vi "PH_StatusHandler.get Status DIM Service.vi"(1 "no link":bool, 2 "typeDescriptor":string, 3 "data":i8[](array[numeric])) -> (0 "Status":T1 items=["no info", "off/false/out", "on/true/in", "Failure", "Alarm", "Status 1", "Status 2", "Status 3"])   [LabVIEW 2014, in "PH_StatusHandler.lvlib"]
doc: "This VI reads out a status service. If \"no link\" is true or the type is not \"S:1\", 0 (no info) is given out."
uses:
  PH_StatusHandler.Status.ctl
  PH_StatusHandler.lvlib
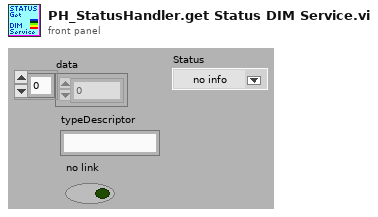
[diagram p1: front panel]
types:
  T1 = typedef "PH_StatusHandler.lvlib/PH_StatusHandler.Status.ctl" = i16
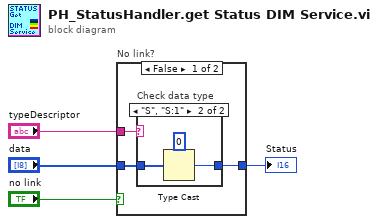
[diagram p0: block diagram]
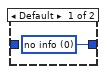
[diagram p2: hidden frame]
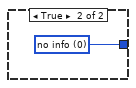
[diagram p3: hidden frame]
diagram:
  n1 = case "No link?" shown="False" "no link" {
    tunnel: [w7 w12] -> w4
    tunnel: "data" -> [w6 _]
    tunnel: "typeDescriptor" -> [w5 _]
    frame False {
      n2 = case "Check data type" shown="\"S\", \"S:1\"" w5 {
        tunnel: [w8 w9] -> w7
        tunnel: w6 -> [_ w10]
        frame Default {
          w8 = T1 0 items=["no info", "off/false/out", "on/true/in", "Failure", "Alarm", "Status 1", "Status 2", "Status 3"] ("Status")
        }
        frame "S", "S:1" {
          n3 = Type Cast(type=i16 0, x=w10) -> (*(type *) &x=w9:i16)
        }
      }
    }
    frame True {
      w12 = T1 0 items=["no info", "off/false/out", "on/true/in", "Failure", "Alarm", "Status 1", "Status 2", "Status 3"] ("Status")
    }
  }
  "Status" <- w4
